vi "Control-DIFuel-Run.vi"(8 "Error In":errorcluster, 11 "DSI Reference":refnum<class "DCM-DSI.lvclass">) -> (0 "Error Out":errorcluster, 3 "DSI Reference":refnum<class "DCM-DSI.lvclass">)   [LabVIEW 2016, in "DSI-RT.lvlib"]
uses:
  DSI-RT.lvlib
  Classes/DCM-DSI/DCM-DSI.lvclass
  Shared/Typedefs/Engine-Channel.ctl
  <vilib>/addons/Software Calibration Management/xSCM/Controls/TLU2D.ctl
  <vilib>/addons/Software Calibration Management/xSCM/Controls/TBL2D.ctl
  Classes/DCM-DSI/Read Channels.vi
  Classes/DCM-DSI/Read EPTx Data.vi
  Classes/DCM-DSI/Write Channels.vi
  <vilib>/addons/Software Calibration Management/xSCM/CalPoint.xnode
  <vilib>/addons/Software Calibration Management/xSCM/ni_scm.dll
  <vilib>/addons/Software Calibration Management/xSCM/SCM-API.lvlib
  Shared/DSI-Shared.lvlib
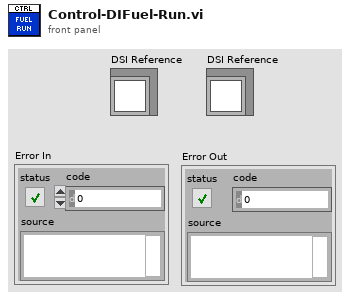
[diagram p1: front panel]
types:
  T1 = typedef "DSI-Shared.lvlib/Engine-Channel.ctl" = cluster{"Name":string, "Unit":string, "Value":sgl}
  T2 = typedef "DCM-DSI.lvclass/Channel.ctl" = cluster{"Name":string, "Unit":string, "Value":sgl}
  T3 = typedef "EPTx - RevA - RT.lvlib/EPTxData.ctl" = cluster{"Sync":bool, "CurrentCAD":sgl, "Speed [RPM]":sgl, "Config":bool, "Rcvg Primary":bool, "Stall":bool, "Overflow":bool, "Ratio Error":bool, "Pattern Error":bool, "Aux Warning":bool, "Watchdog Error":bool}
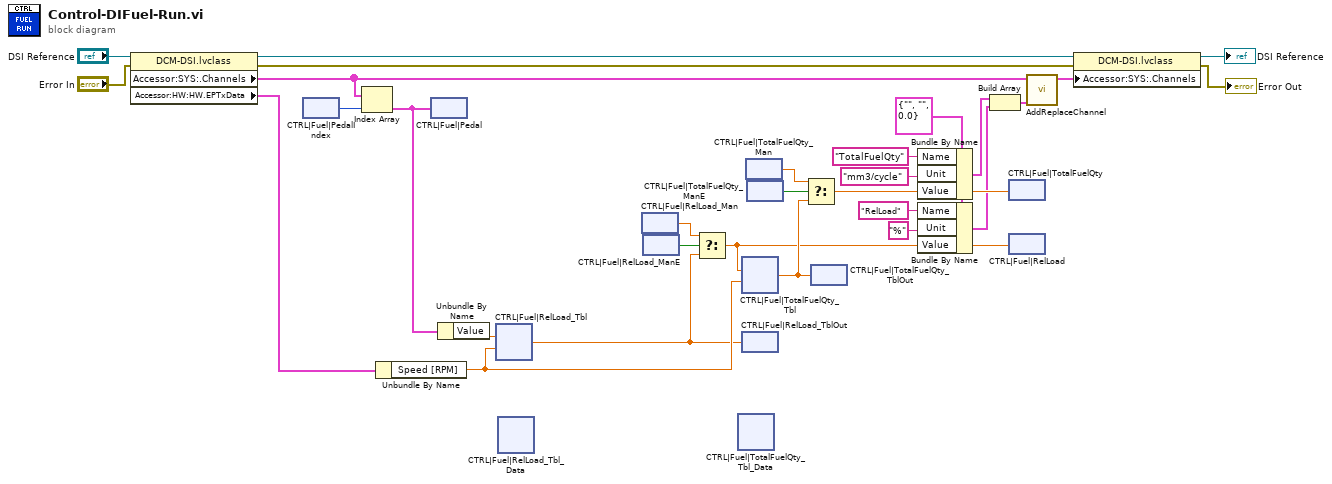
[diagram p0: block diagram]
diagram:
  w3 = T1 {"Name"="", "Unit"="", "Value"=0.0} ("element")
  n1 = property class="DCM-DSI.lvclass"(reference="DSI Reference", error in="Error In") -> (reference out=w27:refnum<class "DCM-DSI.lvclass">, error out=w28:errorcluster, "Accessor:SYS:.Channels"=w7:T2[], "Accessor:HW:HW.EPTxData"=w29:T3)
  n2 = xnode "CTRL|Fuel|PedalIndex"() -> ("Value"=w10:i32)
  n3 = Index Array(array=w7, index=w10) -> (element=w6:T2)
  n4 = Unbundle By Name(w29) -> ("Speed [RPM]"=w18:sgl)
  n5 = xnode "CTRL|Fuel|Pedal"("Value"=w6) -> ()
  n6 = Unbundle By Name(w6) -> ("Value"=w17:sgl)
  n7 = xnode "CTRL|Fuel|RelLoad_Tbl"("Y Index"=w18, "X Index"=w17) -> ("Z"=w15:sgl)
  n8 = xnode "CTRL|Fuel|RelLoad_Tbl_Data"() -> ()  [unwired: 1 out]
  n9 = xnode "CTRL|Fuel|RelLoad_Man"() -> ("Value"=w20:sgl)
  n10 = xnode "CTRL|Fuel|RelLoad_ManE"() -> ("Value"=w19:bool)
  n11 = Select(t=w20, s=w19, f=w15) -> (s? t:f=w1:sgl)
  n12 = xnode "CTRL|Fuel|TotalFuelQty_Tbl_Data"() -> ()  [unwired: 1 out]
  n13 = xnode "CTRL|Fuel|TotalFuelQty_Tbl"("Y Index"=w18, "X Index"=w1) -> ("Z"=w16:sgl)
  n14 = xnode "CTRL|Fuel|RelLoad_TblOut"("Value"=w15) -> ()
  n15 = xnode "CTRL|Fuel|TotalFuelQty_Man"() -> ("Value"=w21:sgl)
  n16 = xnode "CTRL|Fuel|TotalFuelQty_ManE"() -> ("Value"=w22:bool)
  n17 = Select(t=w21, s=w22, f=w16) -> (s? t:f=w8:sgl)
  n18 = xnode "CTRL|Fuel|TotalFuelQty_TblOut"("Value"=w16) -> ()
  n19 = Bundle By Name(cluster=w3, "Name"="TotalFuelQty", "Unit"="mm3/cycle", "Value"=w8) -> (w11:T1)
  n20 = Bundle By Name(cluster=w3, "Name"="RelLoad", "Unit"="%", "Value"=w1) -> (w2:T1)
  n21 = Build Array(w11, w2) -> (w9:T1[])
  n22 = xnode "CTRL|Fuel|TotalFuelQty"("Value"=w8) -> ()
  n23 = xnode "CTRL|Fuel|RelLoad"("Value"=w1) -> ()
  n24 = call "AddReplaceChannel.vi"("Channel In"=w9, "Channels in"=w7) -> ("Channels out"=w12:T1[])  [unwired: 9 in]
  n25 = property class="DCM-DSI.lvclass"(reference=w27, error in=w28, "Accessor:SYS:.Channels"=w12) -> (reference out=→"DSI Reference":refnum<class "DCM-DSI.lvclass">, error out=→"Error Out":errorcluster)
